vi "GFG_core.vi"(0 "Variable Name in":string, 2 "Variant in":variant, 4 "Source VI":string, 5 "error in (no error)":errorcluster, 7 "Action":enum16{"Init", "Set", "Get"}(ring)=enum."Get") -> (13 "Found/Replaced":bool, 14 "Variable Name Out":string, 15 "Data Type Out":T1, 16 "Variant Out":variant, 17 "All Variable Names Out":string[](array[string]), 18 "user event out":refnum<user-event>, 19 "error out":errorcluster)   [LabVIEW 2012]
doc: "This VI represents a functional global variable a.k.a. LV2 Global, which stores any data type as a variant. It was inspired by and adapted from a VI posted on the LabView Idea Exchange (http://forums.ni.com/t5/LabVIEW-Idea-Exchange/Generalized-Functional-Global-GFG/idi-p/1397744)"
uses:
  <vilib>/Utility/VariantDataType/Type.ctl
  <vilib>/Utility/VariantDataType/VariantType.lvlib
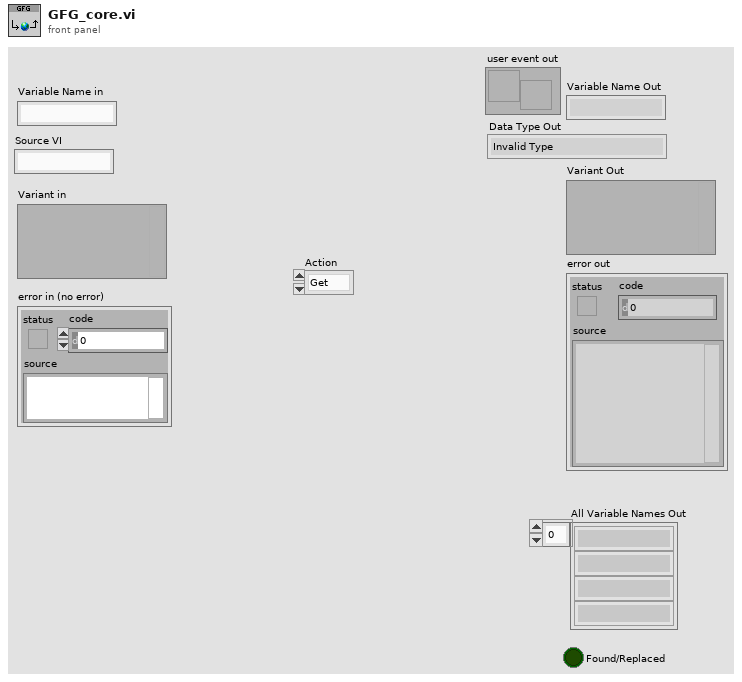
[diagram p1: front panel]
types:
  T1 = typedef "VariantType.lvlib/Type.ctl" = enum8{"Invalid Type", "Void", "I8", "I16", "I32", "I64", "U8", "U16", "U32", "U64", "Single Float", "Double Float", "Extended Float", "Single Complex", "Double Complex", "Extended Complex", "Enum U8", "Enum U16", "Enum U32", "Enum U64", "Single Float With Unit", "Double Float With Unit", "Extended Float With Unit", "Single Complex with Unit", "Double Complex with Unit", "Extended Complex with Unit", "Boolean", "String", "Path", "Picture", "Tag", "Array", "Cluster", "Variant", "LV Variant", "Waveform", "Timestamp", "Digital Waveform", "Digital Data", "ExpressData", "Refnum", "External Data", "VI", "Poly VI", "LabVIEW Class Instance", "Fixed Point"}
  T2 = cluster{"Source VI":string, "Variable Name":string, "Data Type":T1, "Variant":variant}
  T3 = enum16{"open", "replace", "create", "open or create", "replace or create", "replace or create with confirmation"}
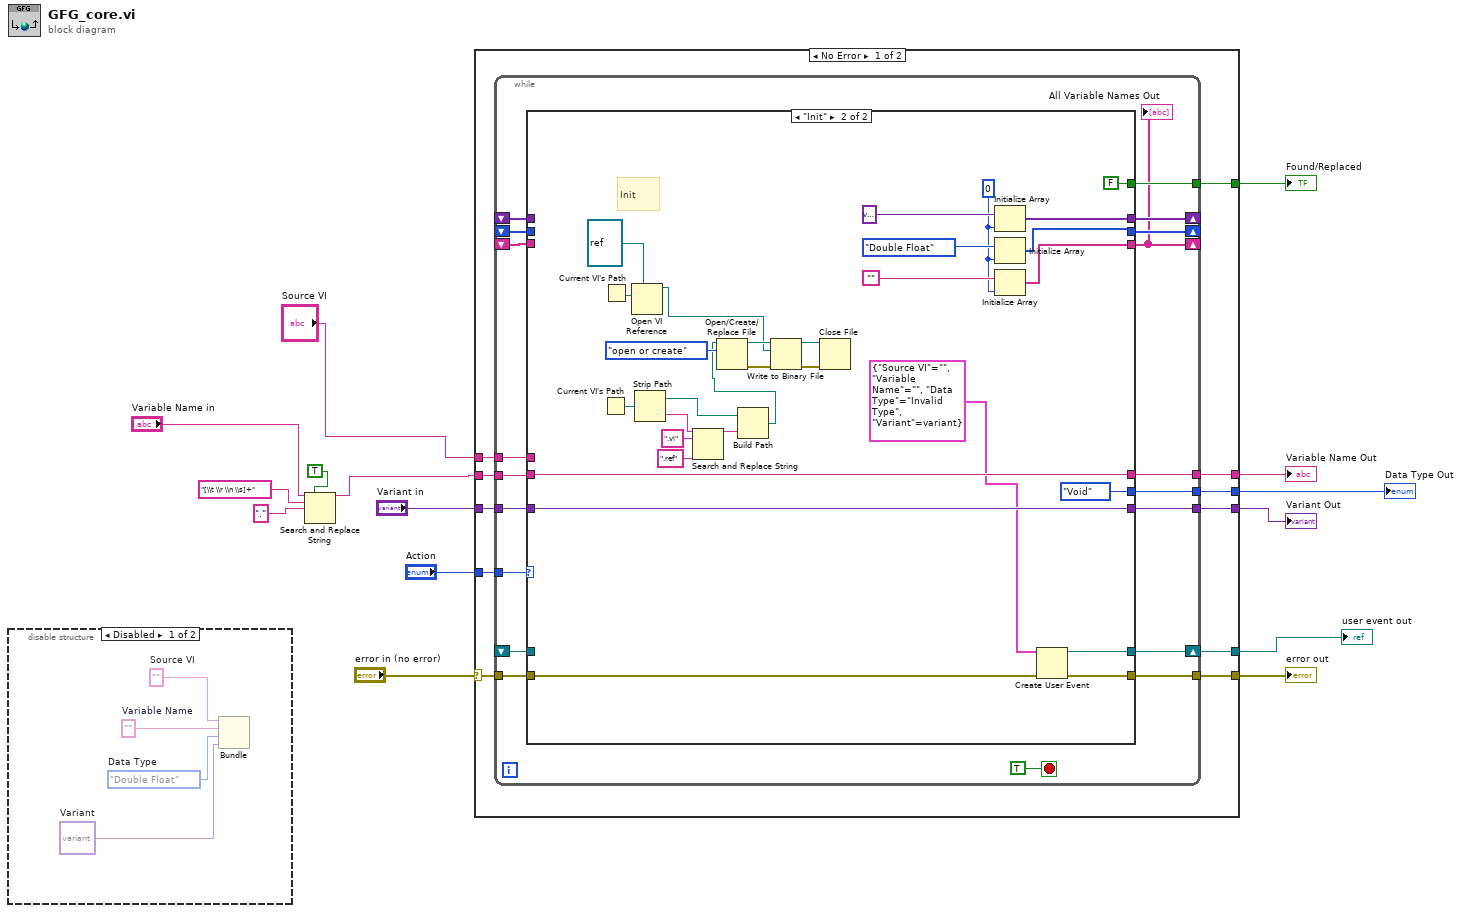
[diagram p0: block diagram]
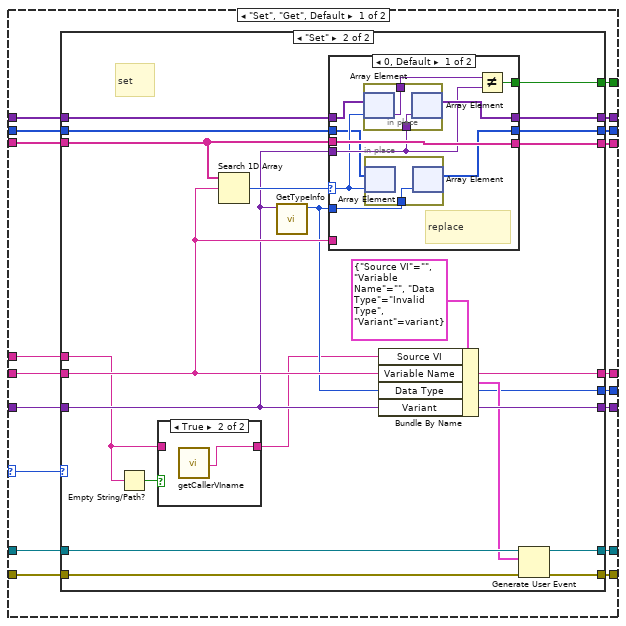
[diagram p3: hidden frame]
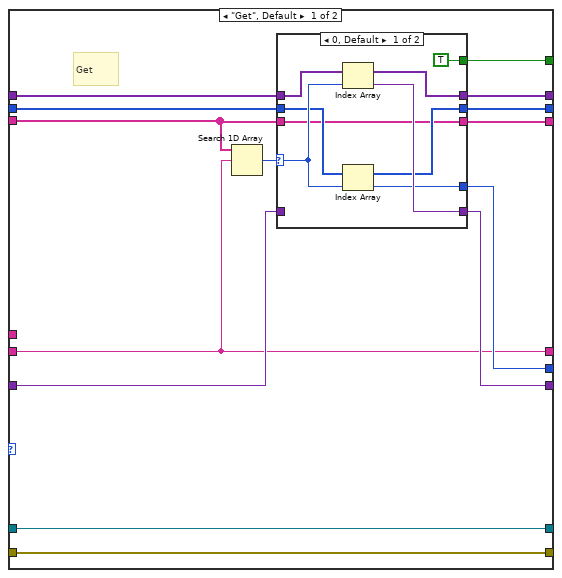
[diagram p4: hidden frame]
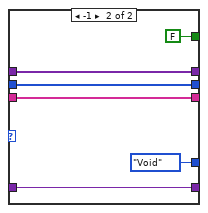
[diagram p5: hidden frame]
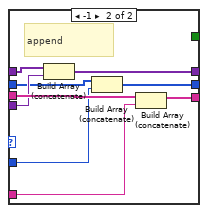
[diagram p7: hidden frame]
diagram:
  n1 = disable-structure shown="Disabled" {
    frame Disabled {
      w16 = variant(bool TRUE)  # Variant
      w18 = ""  # Variable Name
      w19 = ""  # Source VI
      w17 = Type."Double Float"  # Data Type
      n2 = Bundle("Source VI"=w19, "Variable Name"=w18, "Data Type"=w17, "Variant"=w16) -> ()  [unwired: 1 in, 1 out]
    }
    frame Enabled {
    }
  }
  n3 = Search and Replace String(replace all?=TRUE ("replace all? (F)"), input string="Variable Name in", search string="[\\t \\r \\n \\s]+", replace string="." ("replace string (\"\")")) -> (result string=w1:string)  [unwired: 4 in, 3 out]
  n4 = case shown="No Error" "error in (no error)" {
    selector: "error in (no error)" -> [w20 w171]
    tunnel: [w30 w170] -> w15
    tunnel: "Variant in" -> [w29 w170]
    tunnel: [w28 w171] -> w14
    tunnel: w1 -> [w25 w169]
    tunnel: "Source VI" -> [w27 _]
    tunnel: [w26 _] -> w12
    tunnel: [w24 _] -> w8
    tunnel: [w23 _] -> w7
    tunnel: [w22 w169] -> w10
    tunnel: "Action" -> [w21 _]
    frame No Error {
      n5 = while {
        tunnel: [w49] -> w30
        tunnel: w29 -> [w48]
        tunnel: w20 -> [w47]
        tunnel: [w46] -> w28
        tunnel: w25 -> [w44]
        shift-right: [w43] -> w23
        shift-left: _ -> [w42]
        tunnel: w27 -> [w41]
        shift-right: [w33] -> _
        shift-left: _ -> [w40]
        shift-right: [w39] -> _
        shift-left: _ -> [w38]
        tunnel: [w37] -> w26
        shift-right: [w36] -> _
        shift-left: _ -> [w35]
        tunnel: [w34] -> w24
        tunnel: [w32] -> w22
        tunnel: w21 -> [w31]
        stop <- TRUE stop-if-true
        n6 = case shown="\"Init\"" w31 {
          selector: w31 -> [w50 _]
          tunnel: [w60 w164] -> w49
          tunnel: w48 -> [w61 w164]
          tunnel: w47 -> [w65 w168]
          tunnel: [w64 w167] -> w46
          tunnel: w44 -> [w62 w160]
          tunnel: [w66 w159] -> w43
          tunnel: w42 -> [w67 _]
          tunnel: w41 -> [w63 _]
          tunnel: w40 -> [w59 _]
          tunnel: [w58 w166] -> w33
          tunnel: [w56 w163] -> w39
          tunnel: w38 -> [w57 _]
          tunnel: [w55 FALSE] -> w37
          tunnel: [w53 w165] -> w36
          tunnel: w35 -> [w54 _]
          tunnel: [w52 Type."Void" ("Type Enum")] -> w34
          tunnel: [w51 w160] -> w32
          frame "Set", "Get", Default {
            n7 = case shown="\"Set\"" w50 {
              tunnel: w67 -> [w81 w114]
              tunnel: [w81 w100] -> w66
              tunnel: w65 -> [w80 w113]
              tunnel: [w80 w95] -> w64
              tunnel: w63 -> [_ w97]
              tunnel: w62 -> [w70 w104]
              tunnel: w61 -> [w76 w103]
              tunnel: [w75 w103] -> w60
              tunnel: w59 -> [w69 w111]
              tunnel: [w68 w110] -> w58
              tunnel: w57 -> [w78 w109]
              tunnel: [w77 w108] -> w56
              tunnel: [w74 w107] -> w55
              tunnel: w54 -> [w73 w106]
              tunnel: [w72 w105] -> w53
              tunnel: [w71 w99] -> w52
              tunnel: [w70 w104] -> w51
              frame "Get", Default {
                # "Get"
                n8 = Search 1D Array(1D array=w69, element=w70) -> (index of element=w79:i32)  [unwired: 1 in]
                n9 = case shown="0, Default" w79 {
                  selector: w79 -> [w85 _]
                  tunnel: w78 -> [w88 w94]
                  tunnel: [w88 w94] -> w77
                  tunnel: w76 -> [_ w93]
                  tunnel: [w87 w93] -> w75
                  tunnel: [TRUE FALSE] -> w74
                  tunnel: w73 -> [w84 w92]
                  tunnel: [w84 w92] -> w72
                  tunnel: [w83 Type."Void" ("Data Type")] -> w71
                  tunnel: [w82 w91] -> w68
                  tunnel: w69 -> [w82 w91]
                  frame 0, Default {
                    n10 = Index Array(array=w88, index=w85) -> (element=w87:variant)
                    n11 = Index Array(array=w84, index=w85) -> (element=w83:T1)
                  }
                  frame -1 {
                  }
                }
              }
              frame "Set" {
                # "set"
                n12 = Empty String/Path?(string/path=w97) -> (empty?=w98:bool)
                n13 = case shown="True" w98 {
                  tunnel: [w115 w116] -> w96
                  tunnel: w97 -> [w115 _]
                  frame False {
                  }
                  frame True {
                    n14 = call "getCallerVIname.vi"() -> ("VI name"=w116:string)  [unwired: 19 in]
                  }
                }
                n15 = Search 1D Array(1D array=w111, element=w104) -> (index of element=w112:i32)  [unwired: 1 in]
                n16 = call <vilib>:"GetTypeInfo.vi"("Variant"=w103) -> ("Type Enum"=w99:T1)  [unwired: 6 in, 4 out]
                n17 = case shown="0, Default" w112 {
                  selector: w112 -> [w120 _]
                  tunnel: w111 -> [w126 w138]
                  tunnel: [w126 w137] -> w110
                  tunnel: w109 -> [w125 w135]
                  tunnel: w104 -> [_ w136]
                  tunnel: w103 -> [w122 w134]
                  tunnel: [w124 w133] -> w108
                  tunnel: [w121 _] -> w107
                  tunnel: w106 -> [w119 w132]
                  tunnel: w99 -> [w117 w130]
                  tunnel: [w118 w131] -> w105
                  frame 0, Default {
                    # "replace"
                    n18 = in-place {
                      in-place-border: [w129] -> w123
                      in-place-border: w122 -> [w128]
                      n19 = in-place-array #1(w125, w120) -> (w129:variant)
                      n20 = in-place-array #1(w128) -> (w124:variant[])  [unwired: 1 out]
                    }
                    n21 = in-place {
                      in-place-border: w117 -> [w127]
                      n22 = in-place-array #2(w119, w120) -> ()  [unwired: 1 out]
                      n23 = in-place-array #2(w127) -> (w118:T1[])  [unwired: 1 out]
                    }
                    n24 = Not Equal?(x=w123, y=w122) -> (x != y?=w121:bool)
                  }
                  frame -1 {
                    # "append"
                    n25 = Build Array (concatenate)(w135, w134) -> (w133:variant[])
                    n26 = Build Array (concatenate)(w132, w130) -> (w131:T1[])
                    n27 = Build Array (concatenate)(w138, w136) -> (w137:string[])
                  }
                }
                n28 = Bundle By Name(cluster=T2 {"Source VI"="", "Variable Name"="", "Data Type"=enum."Invalid Type", "Variant"=variant} ("output cluster"), "Source VI"=w96, "Variable Name"=w104, "Data Type"=w99, "Variant"=w103) -> (w101:T2)
                n29 = Generate User Event(user event=w114, event data cluster=w101, error in=w113) -> (user event out=w100:refnum<user-event>, error out=w95:errorcluster)
              }
            }
          }
          frame "Init" {
            w155 = 0 ("dimension size")
            # "Init"
            n30 = Current VI's Path() -> (path=w153:path)
            n31 = Current VI's Path() -> (path=w141:path)
            n32 = Open VI Reference(type specifier VI Refnum (for type only)=refnum<vi> refnum, vi path=w141) -> (vi reference=w139:refnum<vi>)  [unwired: 4 in, 1 out]
            n33 = Strip Path(path=w153) -> (stripped path=w149:path, name=w152:string)
            n34 = Search and Replace String(input string=w152, search string=".vi", replace string=".ref" ("replace string (\"\")")) -> (result string=w148:string)  [unwired: 5 in, 3 out]
            n35 = Build Path(base path=w149, name or relative path=w148) -> (appended path=w142:path)
            n36 = Open/Create/Replace File(file path (use dialog)=w142, operation (0:open)=T3."open or create") -> (refnum out=w145:refnum<file>, error out=w144:errorcluster)  [unwired: 4 in, 1 out]
            n37 = Write to Binary File(file (use dialog)=w145, data=w139, error in=w144) -> (refnum out=w146:refnum<file>, error out=w147:errorcluster)  [unwired: 3 in, 1 out]
            n38 = Close File(refnum=w146, error in=w147) -> ()  [unwired: 2 out]
            n39 = Initialize Array(variant ("Variant"), w155) -> (w163:variant[])
            n40 = Initialize Array(Type."Double Float" ("Data Type"), w155) -> (w165:T1[])
            n41 = Initialize Array("" ("Empty String Constant"), w155) -> (w166:string[])
            n42 = Create User Event(user event datatype=T2 {"Source VI"="", "Variable Name"="", "Data Type"=enum."Invalid Type", "Variant"=variant} ("output cluster"), error in=w168) -> (user event=w159:refnum<user-event>, error out=w167:errorcluster)
          }
        }
        "All Variable Names Out" <- w33
      }
    }
    frame Error {
    }
  }
  "Variant Out" <- w15
  "error out" <- w14
  "Found/Replaced" <- w12
  "Variable Name Out" <- w10
  "Data Type Out" <- w8
  "user event out" <- w7
